vi "Stack Rotate.vi"(8 "n":i32, 9 "index":i32, 10 "error in (no error)":errorcluster, 11 "Lua in":refnum<class "Lua.lvclass">) -> (2 "error out":errorcluster, 3 "Lua out":refnum<class "Lua.lvclass">)   [LabVIEW 2020, in "Lua for LabVIEW.lvlib" / "Lua.lvclass"]
doc: "Rotates the stack elements between the valid index idx and the top of the stack. The elements are rotated n positions in the direction of the top, for a positive n, or -n positions in the direction of the bottom, for a negative n. The absolute value of n must not be greater than the size of the slice being rotated. This function cannot be called with a pseudo-index, because a pseudo-index is not an actual stack position."
uses:
  Lua.lvclass
  Lua.lvclass/Lua.ctl
  lib/lua.dll/lua.dll.lvlib
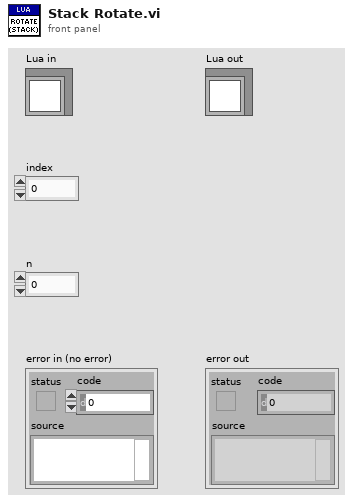
[diagram p1: front panel]
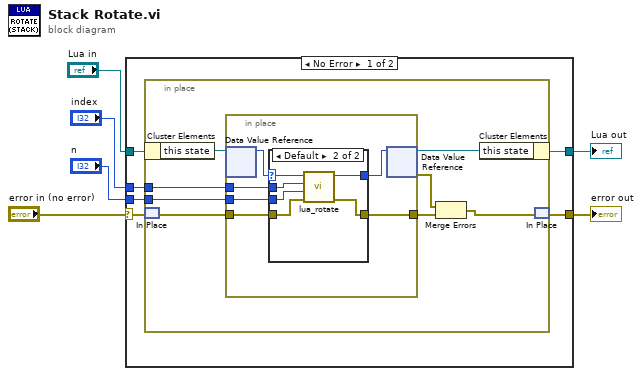
[diagram p0: block diagram]
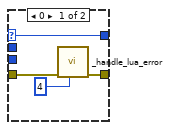
[diagram p2: hidden frame]
diagram:
  n1 = case shown="No Error" "error in (no error)" {
    selector: "error in (no error)" -> [w9 w38]
    tunnel: [w10 w38] -> w5
    tunnel: [w11 w37] -> w3
    tunnel: "Lua in" -> [w12 w37]
    tunnel: "index" -> [w8 _]
    tunnel: "n" -> [w7 _]
    frame No Error {
      n2 = in-place {
        in-place-border: w8 -> [w19]
        in-place-border: w7 -> [w18]
        n3 = in-place-cluster #1(w12) -> ("this state"=w17:refnum<data-value>)
        n4 = in-place-match #2(w9) -> (w20:errorcluster)
        n5 = in-place {
          in-place-border: w20 -> [w26]
          in-place-border: w19 -> [w25]
          in-place-border: w18 -> [w24]
          in-place-border: [w21] -> w14
          n6 = in-place-dvr #3(w17) -> (w23:u64)  [unwired: 1 out]
          n7 = case shown="Default" w23 {
            selector: w23 -> [w30 w35]
            tunnel: [w30 w36] -> w22
            tunnel: w26 -> [w27 w34]
            tunnel: [w28 w33] -> w21
            tunnel: w25 -> [_ w32]
            tunnel: w24 -> [_ w31]
            frame 0 {
              n8 = call "_handle_lua_error.vi"("lua status"=4 ("lua_load errcode"), "error in (no error)"=w27) -> ("error out"=w28:errorcluster)  [unwired: 9 in]
            }
            frame Default {
              n9 = call "lua_rotate.vi"("error in (no error)"=w34, "n"=w31, "index"=w32, "lua_state_p"=w35) -> ("error out"=w33:errorcluster, "lua_state_p out"=w36:u64)  [unwired: 6 in]
            }
          }
          n10 = in-place-dvr #3(w22) -> (w16:refnum<data-value>, w15:errorcluster)
        }
        n11 = Merge Errors(w15, w14) -> (w13:errorcluster)
        n12 = in-place-cluster #1("this state"=w16) -> (w11:refnum<class "Lua.lvclass">)
        n13 = in-place-match #2(w13) -> (w10:errorcluster)
      }
    }
    frame Error {
    }
  }
  "error out" <- w5
  "Lua out" <- w3
